vi "MAT_Master.vi"(11 "Settings in":T3={"Name of test"="", "Date"=timestamp(0 s since 1904-01-01), "Location"="", "Template"="", "Soundcard"="", "resolution"=32, "Sampling rate"=48000, "Ch1 Gain "=25.0, "Ch2 Gain"=10.0, "Sample time (s)"=0.3, "Pre-trigger (s)"=0.01, "Hammer Threshold"=10.0, "Positions"=12, "Taps/Position"=5, "Set Names"="", "Freq resolution"=10.0, "Hammer cutoff"=0.0, "Mic cutoff"=0.0, "Double bounce "=0.0, "Hammer Cal"=10.0, "dB Offset"=0.0, "Accel Cal"=10.0, "Vibrometer Cal"=0.0, "Mic Cal"=0.0, "Output"=2, "Voltage Cal"=1.0, "Vibrometer Port"="ASRL27::INSTR", "Range"=4, "High Pass"=2, "Bandwidth"=4, "X Range"=[], "Y Range"=[], "dB Spread"=0.0, "Trigger"=0, "Ch_1"=25, "Ch_2"=25, "flip?"=FALSE, "60Hz"=FALSE, "Time offset"=0.0, "Piezo Cal"=1.0, "Default Notes"=""} {"Ch_2" min=1 step=1; "Ch_1" min=1 max=100 step=1; "Trigger" items=["Hammer (force)", "Self-tap", "Spacebar"]; "Bandwidth" items=["1 kHz"=1, "5 kHz"=5, "10 kHz"=10, "25 kHz"=25, "50 kHz"=50, "100 kHz"=100]; "High Pass" items=["Off", "13 Hz", "104 Hz"]; "Range" items=["10 mm/s"=1, "20 mm/s"=2, "50 mm/s"=5, "100 mm/s"=10, "200 mm/s"=20, "500 mm/s"=50, "1 m/s"=100, "2 m/s"=200]; "Output" items=["Accelerometer", "Speed (from acceleration)", "Microphone", "Vibrometer", "Piezo"]; "Voltage Cal" format="%#_13g"; "Ch2 Gain" format="%#_13g"; "Ch1 Gain" format="%#_13g"; "Double bounce" min=0.0; "Mic cutoff" min=0.0 format="%#_4g"; "Hammer cutoff" min=0.0 format="%#_4g"; "Freq resolution" min=0.0; "Pre-trigger (s)" format="%#_13g"; "Date" format="%<%H:%M\n%d/%m/%y>T"; "resolution" items=["16 bit"=16, "24 bit"=24, "32 bit"=32]; "Sampling rate" items=["22050 samp/s"=22050, "44100 samp/s"=44100, "48000 samp/s"=48000]}) -> ()   [LabVIEW 2022 SP3]
uses:
  PreferencesControl.ctl
  Subs/miDataType.ctl
  <vilib>/Utility/error.llb/Trim Whitespace One-Sided.vi
panel:
  in  "Tab Control":enum32{"Intro", "Params", "Settings", "Saving"}(tab)
  in  "Save Button":bool
  in  "Instrument Name":string(combo)
  in  "Settings":bool
  in  "MAT Path":path
  out "FRF":cluster{"x0":dbl, "df":dbl, dbl[]}[](graph)
  in  "Back":bool
  out "Title":string
  out "Array":T2(array[cluster])
  out "Graph":cluster{dbl, dbl, "Magnitude":dbl[]}[](graph)
  out "dt2":dbl[](array[numeric])
  out "fsampling":dbl
  out "npts":dbl
  out "tfun":dbl
  out "Complex":cluster{dbl, dbl, "complex":cdb[]}[](array[cluster])
  out "Slide":u8(slide) scale=0.0..100.0
  out "Info":string
  # "Welcome To The MAT File Translator"
  # "This will translate a MAT file of Woodhouse Layout (and read the various headers)"
  # "1. Select a file\nHit the folder button or drag a file on"
  # "2. Translate the data\nMake sure the data looks good"
  # "3. Save as an instrument\nAdd to an existing or create a new instrument"
  # "4. Repeat or Close\nOpen a new file or close the window"
  # "time chan    spect    sonogram"
  # "Hz"
  # "dB"
  # "dB"
  # "sec"
  # "sec"
  # "mV/Pa"
  # "mV/m/s2"
  # "mV/mm/s"
  # "V/N"
  # "sec"
  # "sec"
  # "mV/N"
  # "a.u."
  # "a.u."
  # "sec"
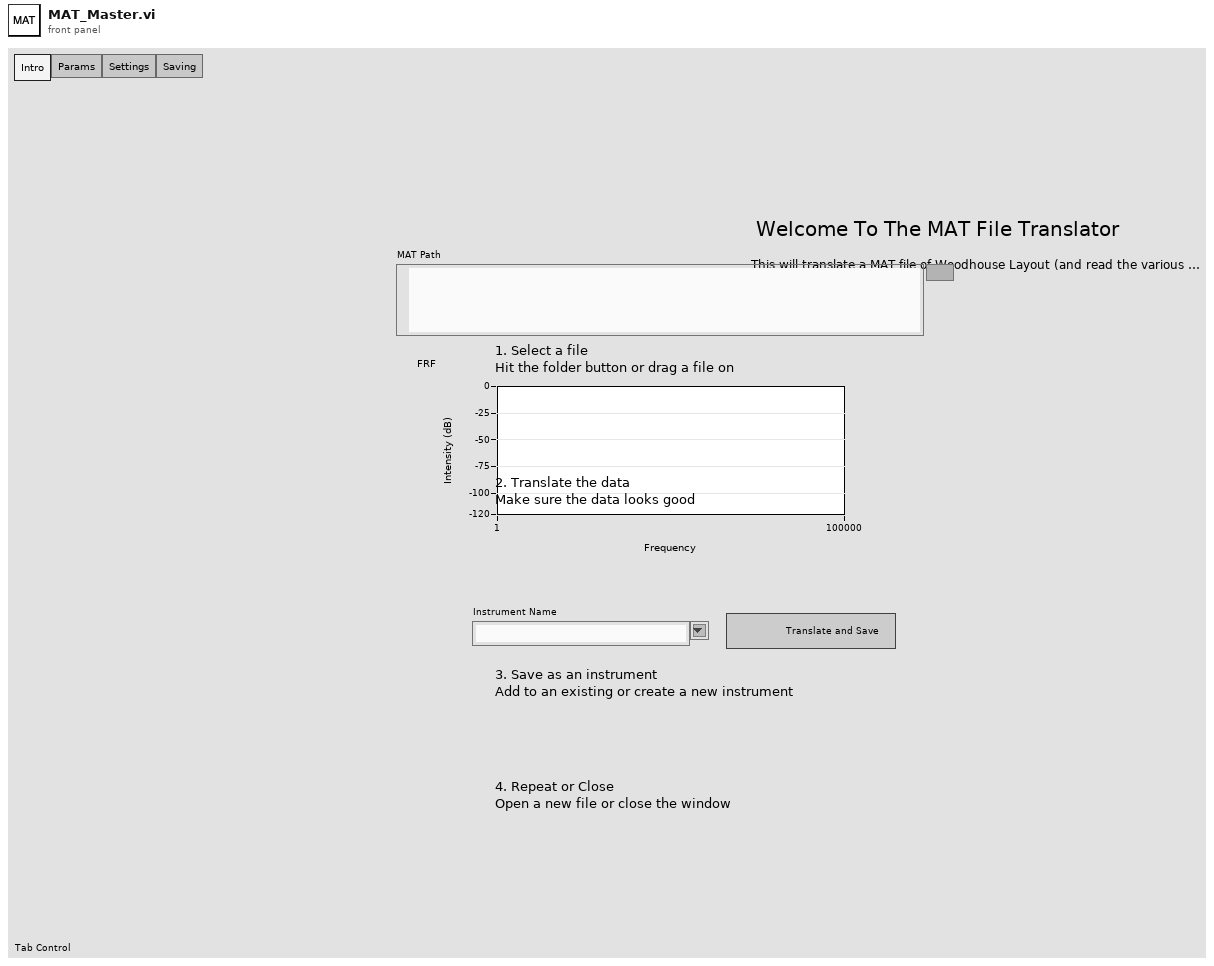
[diagram p1: front panel]
types:
  T1 = typedef "miDataType.ctl" = enum16{"illegal", "miINT8", "miUINT8", "miINT16", "miUINT16", "miINT32", "miUINT32", "miSINGLE", "--", "miDOUBLE", "---", "----", "miINT64", "miUINT64", "miMATRIX", "miCOMPRESSED", "miUTF8", "miUTF16", "miUTF32", "udefined"}
  T2 = cluster{"Array Flags":cluster{"Data Type":T1, "# bytes":u32, "data":string}, "Dimensions Array":cluster{"Data Type":T1, "# bytes":u32, "data":string}, "Array Name":cluster{"Data Type":T1, "# bytes":u32, "data":string}, cluster{"complex":bool, "global":bool, "logical":bool}, "Data":dbl[][]}[]
  T3 = typedef "PreferencesControl.ctl" = cluster{"Name of test":string, "Date":timestamp, "Location":string, "Template":string, "Soundcard":string, "resolution":u16, "Sampling rate":u16, "Ch1 Gain ":dbl, "Ch2 Gain":dbl, "Sample time (s)":dbl, "Pre-trigger (s)":dbl, "Hammer Threshold":dbl, "Positions":i16, "Taps/Position":i16, "Set Names":string, "Freq resolution":dbl, "Hammer cutoff":dbl, "Mic cutoff":dbl, "Double bounce ":dbl, "Hammer Cal":dbl, "dB Offset":dbl, "Accel Cal":dbl, "Vibrometer Cal":dbl, "Mic Cal":dbl, "Output":u16, "Voltage Cal":dbl, "Vibrometer Port":refnum<visa-resource-name>, "Range":u16, "High Pass":u16, "Bandwidth":u16, "X Range":cluster{"Minimum":dbl, "Maximum":dbl, "Increment":dbl, "Minor Increment":dbl, "Start":dbl}[], "Y Range":cluster{"Minimum":dbl, "Maximum":dbl, "Increment":dbl, "Minor Increment":dbl, "Start":dbl}[], "dB Spread":dbl, "Trigger":u16, "Ch_1":u8, "Ch_2":u8, "flip?":bool, "60Hz":bool, "Time offset":dbl, "Piezo Cal":dbl, "Default Notes":string}
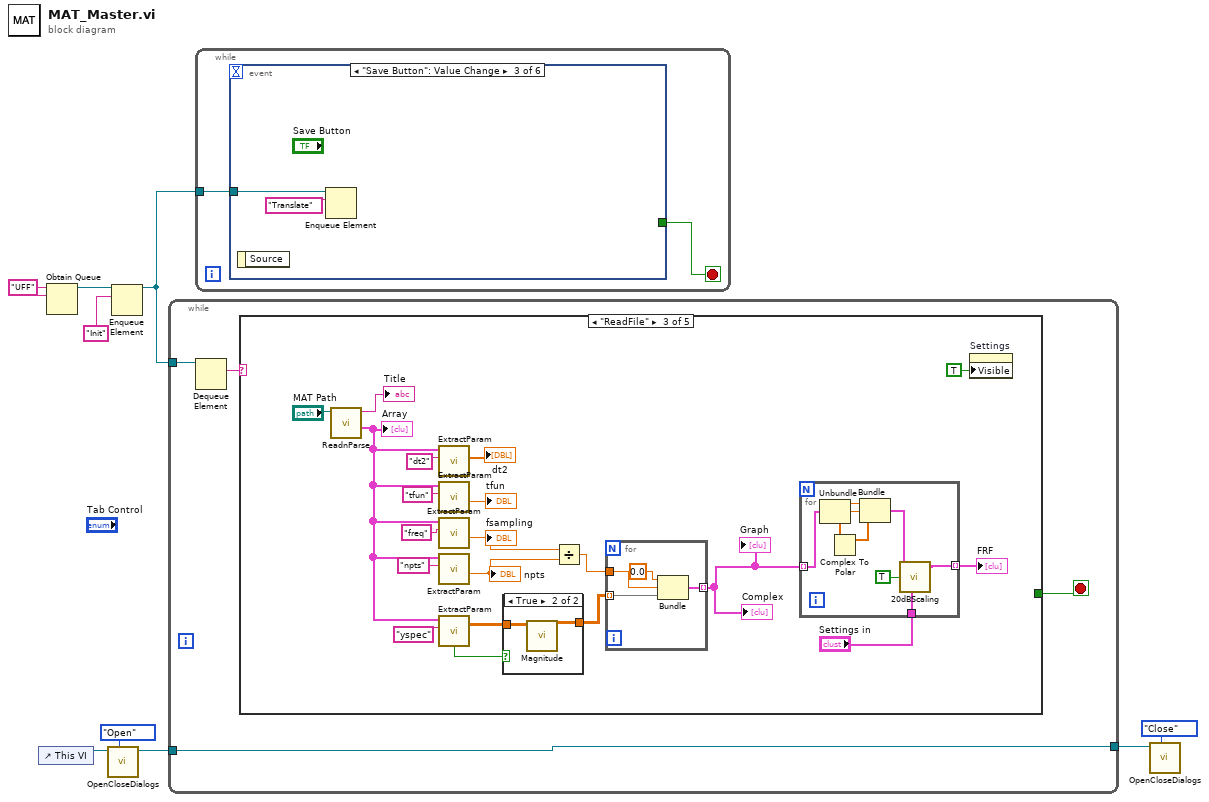
[diagram p0: block diagram]
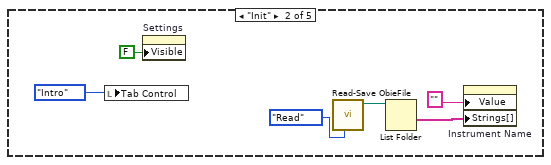
[diagram p3: hidden frame]
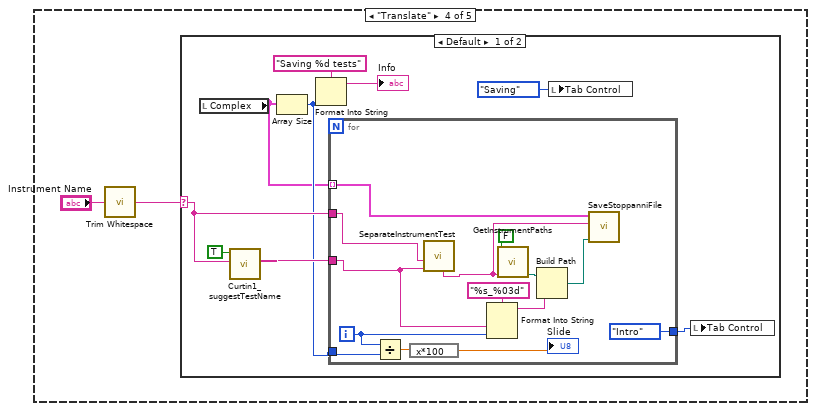
[diagram p5: hidden frame]
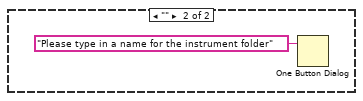
[diagram p6: hidden frame]
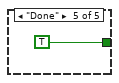
[diagram p7: hidden frame]
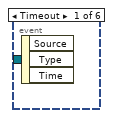
[diagram p8: hidden frame]
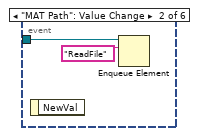
[diagram p9: hidden frame]
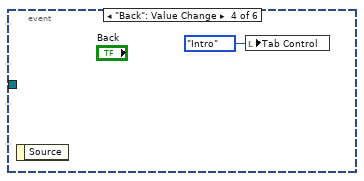
[diagram p10: hidden frame]
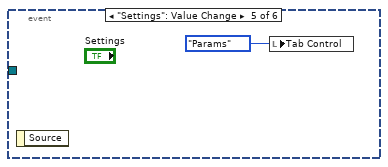
[diagram p11: hidden frame]
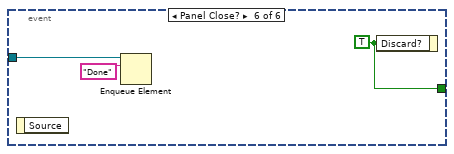
[diagram p12: hidden frame]
diagram:
  w9 = "UFF" ("name (unnamed)")
  n1 = control-ref of="This VI"() -> (w4:refnum<vi>)
  n2 = Obtain Queue(name (unnamed)=w9, element data type=w9) -> (queue out=w7:refnum<queue>)  [unwired: 3 in, 2 out]
  n3 = call "OpenCloseDialogs.vi"("Task"=enum16{"Open", "Close"}."Open", "VI in"=w4) -> ("VI out"=w1:refnum<vi>)  [unwired: 8 in, 1 out]
  n4 = Enqueue Element(queue=w7, element="Init") -> (queue out=w6:refnum<queue>)  [unwired: 2 in, 2 out]
  n5 = while {
    tunnel: w6 -> [w13]
    tunnel: [w10] -> w2
    tunnel: w1 -> [w10]
    stop <- w11 stop-if-true
    n6 = Dequeue Element(queue=w13) -> (element=w12:string)  [unwired: 2 in, 3 out]
    n7 = case shown="\"ReadFile\"" w12 {
      tunnel: [_ _ _ _ TRUE ("Discard?")] -> w11
      frame Default {
      }
      frame "Init" {
        n8 = local write "Tab Control"(enum32{"Intro", "Params", "Settings"}."Intro" ("Tab Control")) -> ()
        n9 = property on="Settings" class="Bool"("Visible"=FALSE) -> ()  [unwired: 2 in, 2 out]
        n10 = call "Read-Save ObieFile.vi"("Task"=enum16{"Save", "Read"}."Read") -> ("DataPath Out"=w16:path)  [unwired: 8 in, 2 out]
        n11 = List Folder(path=w16) -> (folder names=w15:string[])  [unwired: 3 in, 3 out]
        n12 = property on="Instrument Name" class="CmbBox"("Value"="" ("Value (Signaling)"), "Strings[]"=w15) -> ()  [unwired: 2 in, 2 out]
      }
      frame "ReadFile" {
        n13 = call "ReadnParse.vi"("MAT Path"="MAT Path") -> ("Array"=w28:T2, "Title"=→"Title":string)  [unwired: 7 in, 2 out]
        "Array" <- w28
        n14 = call "ExtractParam.vi"("String"="dt2", "Array"=w28) -> ("1st Col"=→"dt2":dbl[])  [unwired: 5 in, 4 out]
        n15 = call "ExtractParam.vi"("String"="tfun", "Array"=w28) -> ("1st pt"=→"tfun":dbl)  [unwired: 5 in, 4 out]
        n16 = call "ExtractParam.vi"("String"="freq", "Array"=w28) -> ("1st pt"=w26:dbl)  [unwired: 5 in, 4 out]
        "fsampling" <- w26
        n17 = call "ExtractParam.vi"("String"="npts", "Array"=w28) -> ("1st pt"=w27:dbl)  [unwired: 5 in, 4 out]
        "npts" <- w27
        n18 = call "ExtractParam.vi"("String"="yspec", "Array"=w28) -> ("Data"=w22:dbl[][], "complex"=w20:bool)  [unwired: 5 in, 3 out]
        n19 = case shown="True" w20 {
          tunnel: w22 -> [w40 w42]
          tunnel: [w40 w41] -> w21
          frame False {
          }
          frame True {
            n20 = call "Magnitude.vi"("Data in"=w42) -> ("complex"=w41:cdb[][])  [unwired: 8 in, 2 out]
          }
        }
        n21 = Divide(x=w26, y=w27) -> (x/y=w34:dbl)
        n22 = for {
          tunnel: w34 -> [w53]
          tunnel: w21 -> [w52] mode=indexing
          tunnel: [w55] -> w23 mode=indexing
          n23 = Bundle(0.0, w53, "complex"=w52) -> (w55:cluster{dbl, dbl, "complex":cdb[]})  [unwired: 1 in]
        }
        "Graph" <- w23
        "Complex" <- w23
        n24 = for {
          tunnel: "Settings in" -> [w50]
          tunnel: [w49] -> w24 mode=indexing
          tunnel: w23 -> [w44] mode=indexing
          n25 = Unbundle(w44) -> (w48:dbl, w47:dbl, "complex"=w46:cdb[])
          n26 = Complex To Polar(r * e^(i*theta)=w46) -> (r=w45:dbl[])  [unwired: 1 out]
          n27 = Bundle(w48, w47, w45) -> (w43:cluster{dbl, dbl, dbl[]})  [unwired: 1 in]
          n28 = call "20dBScaling.vi"("Average FRF in"=w43, "dB?"=TRUE, "Settings"=w50) -> ("Average FRF out"=w49:cluster{"x0":dbl, "df":dbl, dbl[]})  [unwired: 3 in, 1 out]
        }
        "FRF" <- w24
        n29 = property on="Settings" class="Bool"("Visible"=TRUE) -> ()  [unwired: 2 in, 2 out]
      }
      frame "Translate" {
        n30 = call <vilib>:"Trim Whitespace.vi"("string"="Instrument Name") -> ("trimmed string"=w56:string)  [unwired: 1 in]
        n31 = case shown="Default" w56 {
          selector: w56 -> [w65 _]
          frame Default {
            n32 = local read "Complex"() -> (w58:cluster{dbl, dbl, "complex":cdb[]}[])
            n33 = call "Curtin1_suggestTestName.vi"("instrument"=w65, "Build?"=TRUE) -> ("Suggested Test"=w63:string)  [unwired: 9 in]
            n34 = Array Size(array=w58) -> (size(s)=w61:i32)
            n35 = Format Into String(format string="Saving %d tests", w61) -> (resulting string=→"Info":string)  [unwired: 2 in, 1 out]
            n36 = for {
              tunnel: w65 -> [w76]
              tunnel: w63 -> [w73]
              tunnel: w61 -> [w71]
              tunnel: [enum32{"Intro", "Params", "Settings", "Saving"}."Intro" ("Tab Control")] -> w59
              tunnel: w58 -> [w67] mode=indexing
              i -> [w72]
              n37 = Divide(x=w72, y=w71) -> (x/y=w70:dbl)
              n38 = expression code="x*100"(w70) -> (→"Slide":dbl)
              n39 = call "SeparateInstrumentTest.vi"("test in"=w73, "Instrument in"=w76) -> ("Instrument -- test out"=w79:string)  [unwired: 5 in, 4 out]
              n40 = Format Into String(format string="%s_%03d", w73, w72) -> (resulting string=w74:string)  [unwired: 2 in, 1 out]
              n41 = call "GetInstrumentPaths.vi"("Instrument"=w79, "Build?"=FALSE) -> ("Path To Raw Folder"=w78:path)  [unwired: 5 in, 4 out]
              n42 = Build Path(base path=w78, name or relative path=w74) -> (appended path=w77:path)
              n43 = call "SaveStoppanniFile.vi"("Last Path"=w77, "Inst:Test Name"=w79, "Complex FRF"=w67) -> ()  [unwired: 8 in, 1 out]
            }
            n44 = local write "Tab Control"(enum32{"Intro", "Params", "Settings", "Saving"}."Saving" ("Tab Control")) -> ()
            n45 = local write "Tab Control"(w59) -> ()
          }
          frame "" {
            n46 = One Button Dialog(message="Please type in a name for the instrument folder") -> ()  [unwired: 1 in, 1 out]
          }
        }
      }
      frame "Done" {
      }
    }
  }
  n47 = while {
    tunnel: w6 -> [w84]
    stop <- w83 stop-if-true
    n48 = event shown="[2] \"Save Button\": Value Change" {
      selector: _ -> [_ _ _ _ _ _]
      dyn-events: _ -> [_ _ _ _ _ _]
      timeout: _ -> [_ _ _ _ _ _]
      tunnel: w84 -> [_ w86 w88 _ _ w91]
      tunnel: [_ _ _ _ _ w93] -> w83
      event Timeout {
        n49 = event-data() -> ()  [unwired: 1 in, 3 out]
      }
      event "MAT Path": Value Change {
        n50 = event-data() -> ()  [unwired: 1 in, 1 out]
        n51 = Enqueue Element(queue=w86, element="ReadFile") -> ()  [unwired: 2 in, 3 out]
      }
      event "Save Button": Value Change {
        n52 = event-data() -> ()  [unwired: 1 in, 1 out]
        n53 = Enqueue Element(queue=w88, element="Translate") -> ()  [unwired: 2 in, 3 out]
      }
      event "Back": Value Change {
        n54 = event-data() -> ()  [unwired: 1 in, 1 out]
        n55 = local write "Tab Control"(enum32{"Intro", "Params", "Settings"}."Intro" ("Tab Control")) -> ()
      }
      event "Settings": Value Change {
        n56 = event-data() -> ()  [unwired: 1 in, 1 out]
        n57 = local write "Tab Control"(enum32{"Intro", "Params", "Settings"}."Params" ("Tab Control")) -> ()
      }
      event Panel Close? {
        w93 = TRUE ("Discard?")
        n58 = event-data() -> ()  [unwired: 1 in, 1 out]
        n59 = Enqueue Element(queue=w91, element="Done") -> ()  [unwired: 2 in, 3 out]
        n60 = event-data("Discard?"=w93) -> ()  [unwired: 1 in, 1 out]
      }
    }
  }
  n61 = call "OpenCloseDialogs.vi"("Task"=enum16{"Open", "Close"}."Close", "VI in"=w2) -> ()  [unwired: 8 in, 2 out]
